vi "Log to Disk.vi"() -> ()   [LabVIEW 2014]
uses:
  CAN/MC/MC Temp 1.ctl
panel:
  in  "stop":bool
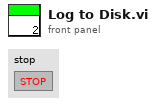
[diagram p1: front panel]
types:
  T1 = enum16{"open", "open or create", "create or replace", "create", "open (read-only)"}
  T2 = typedef "MC Temp 1.ctl" = cluster{"IGBT A (C)":dbl, "IGBT B (C)":dbl, "IGBT C (C)":dbl, "Gate Driver (C)":dbl}
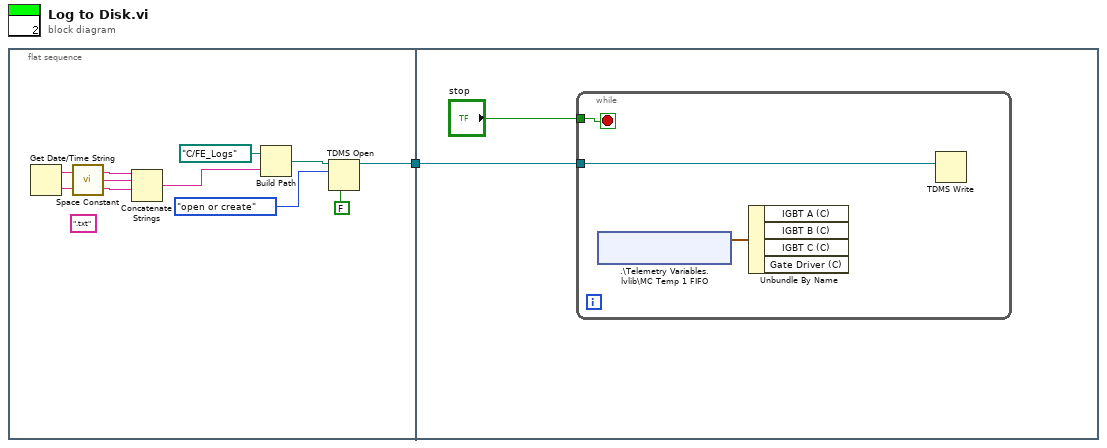
[diagram p0: block diagram]
diagram:
  n1 = flat-sequence {
    tunnel: [w2] -> w1
    tunnel: w1 -> [w11]
    frame #0 {
      (unwired) ".txt" ("string")
      n2 = Get Date/Time String() -> (date string=w7:string, time string=w9:string)  [unwired: 3 in]
      n3 = call <vilib>:"Space Constant.vi"() -> ("String"=w8:string)
      n4 = Concatenate Strings(w7, w8, w9) -> (w10:string)  [unwired: 1 in]
      n5 = Build Path(base path=path "C:/FE_Logs", name or relative path=w10) -> (appended path=w5:path)
      n6 = TDMS Open(6:FALSE ("disable buffering? (T)"), 10:T1."open or create" ("operation (0:open)"), 11:w5) -> (3:w2:refnum<k34>)  [unwired: 4 in, 1 out]
    }
    frame #1 {
      n7 = while {
        tunnel: "stop" -> [w16]
        tunnel: w11 -> [w15]
        stop <- w16 stop-if-true
        n8 = shared-variable ".\\Telemetry Variables.lvlib\\MC Temp 1 FIFO"() -> (w14:T2)  [unwired: 1 in, 2 out]
        n9 = Unbundle By Name(w14) -> ()  [unwired: 4 out]
        n10 = TDMS Write(0:w15) -> (9:w13:waveform(dbl)[])  [unwired: 4 in, 4 out]
      }
    }
  }
